vi "Obtain Message Queue (enum).vi"(8 "error in (no error)":errorcluster, 10 "Message":T1) -> (0 "error out":errorcluster, 3 "queue out":refnum<queue>)   [LabVIEW 2018, in "Message Queue.lvlib"]
doc: "Create a queue with the Message Cluster data type."
uses:
  Message Queue.lvlib
  Message (enum).ctl
  Message Cluster (enum).ctl
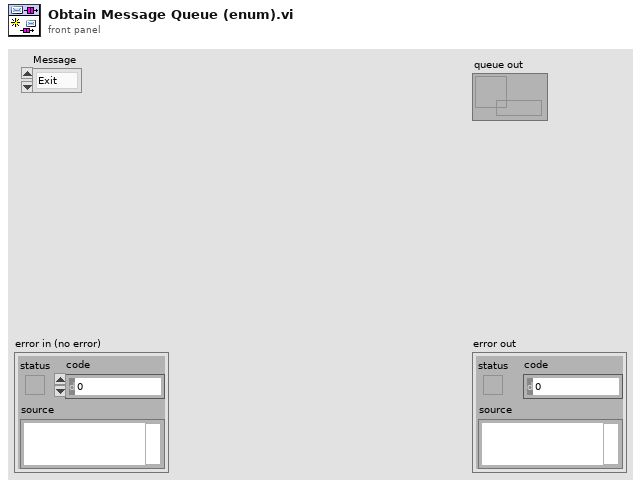
[diagram p1: front panel]
types:
  T1 = typedef "Message Queue.lvlib/Message (enum).ctl" = enum16{"Exit"}
  T2 = typedef "Message Queue.lvlib/Message Cluster (enum).ctl" = cluster{"Message":T1, "Message Data":variant}
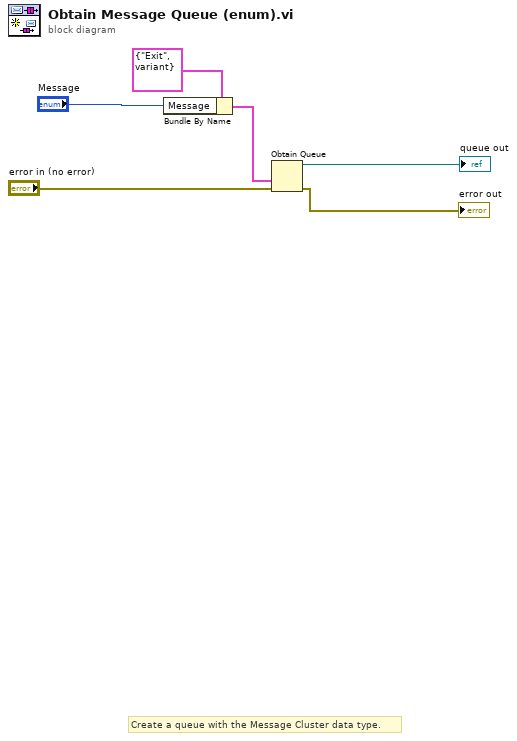
[diagram p0: block diagram]
diagram:
  # "Create a queue with the Message Cluster data type."
  n1 = Bundle By Name(cluster=T2 {"Message"=enum."Exit", "Message Data"=variant} ("Message Cluster"), "Message"="Message") -> (w2:T2)
  n2 = Obtain Queue(create if not found? (T)=w2, error in (no error)="error in (no error)") -> (queue out=→"queue out":refnum<queue>, error out=→"error out":errorcluster)  [unwired: 3 in, 1 out]
